vi "Move_Piezo.vi"(5 "Piezo":u16(ring)=1 items=["X (AO0)", "Y (AO1)", "Z (AO2)", "V (AO3)", "V2 (AO4)"], 7 "Movement Speed (µm/s)":dbl=5.0 min=0.0 max=20.0, 11 "Position (µm) (or V)":dbl min=-10.0 max=1000.0) -> ()   [LabVIEW 2023]
uses:
  Sub_Vi/TypeDefs/Settings.ctl
  Sub_Vi/TypeDefs/WayPointCluster.ctl
  Sub_Vi/TypeDefs/ChangeOnFly.ctl
  Settings.vi
panel:
  in  "stop":bool
  in  "WayPointCluster":T1
  in  "SettingsCluster":T2={"Sample Rate (us)"=1, "Samples Per Data Point (int, power of 2)"=1000, "DistanceToBulk (um)"=-1.0, "HoldTimeScaler"=1, "SaveData"=FALSE, "DistanceToBulk (um) 2"=-1.0, "DistanceToBulk (um) 3"=-1.0}
  # "Settings"
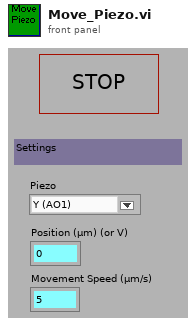
[diagram p1: front panel]
types:
  T1 = typedef "WayPointCluster.ctl" = cluster{"X (um)":dbl[], "Y (um)":dbl[], "Z (um)":dbl[], "V (V)":dbl[], "X Velocity (um s-1)":dbl[], "Y Velocity (um s-1)":dbl[], "Z Velocity (um s-1)":dbl[], "V Velocity (V s-1)":dbl[], "FeedBack Type (enum)":u16[], "Move X (boolean)":bool[], "Move Y (boolean)":bool[], "Move Z (boolean)":bool[], "Move V (boolean)":bool[], "Jump V (boolean)":bool[], "Hold (boolean)":bool[], "Hold Time":u32[], "V2 (V)":dbl[], "Move V2":bool[], "V2 Velocity (V s-1)":dbl[], "Jump V2 (boolean)":bool[], "Update z Position delta (ms)":i16[], "Hold Feedback1":bool[], "Move Z PicoMotor":bool[], " Z PicoMotor Direction":bool[], "DIO0":bool[]}
  T2 = typedef "Settings.ctl" = cluster{"Sample Rate (us)":u32, "Samples Per Data Point (int, power of 2)":i16, "DistanceToBulk (um)":dbl, "HoldTimeScaler":u64, "SaveData":bool, "DistanceToBulk (um) 2":dbl, "DistanceToBulk (um) 3":dbl}
  T3 = typedef "ChangeOnFly.ctl" = cluster{"Stop (boolean)":refnum<vi>, "Pause (boolean)":refnum<vi>, "EndCurrentLine (boolean)":refnum<vi>, "max movement per update step (Interger, nm)":refnum<vi>, "P (float, arb)":refnum<vi>, "Feedback set point (double, Amps)":refnum<vi>, "Voltage (double, V)":refnum<vi>, "Feedback set point 2 (double, Amps)":refnum<vi>, "Stop on Greater Than 2? (boolean)":refnum<vi>, "Stop on Greater Than? (boolean)":refnum<vi>, "Voltage 2 (double, V)":refnum<vi>, "Feedback Type (enum)":refnum<vi>, "Feedback Type 2 (enum)":refnum<vi>}
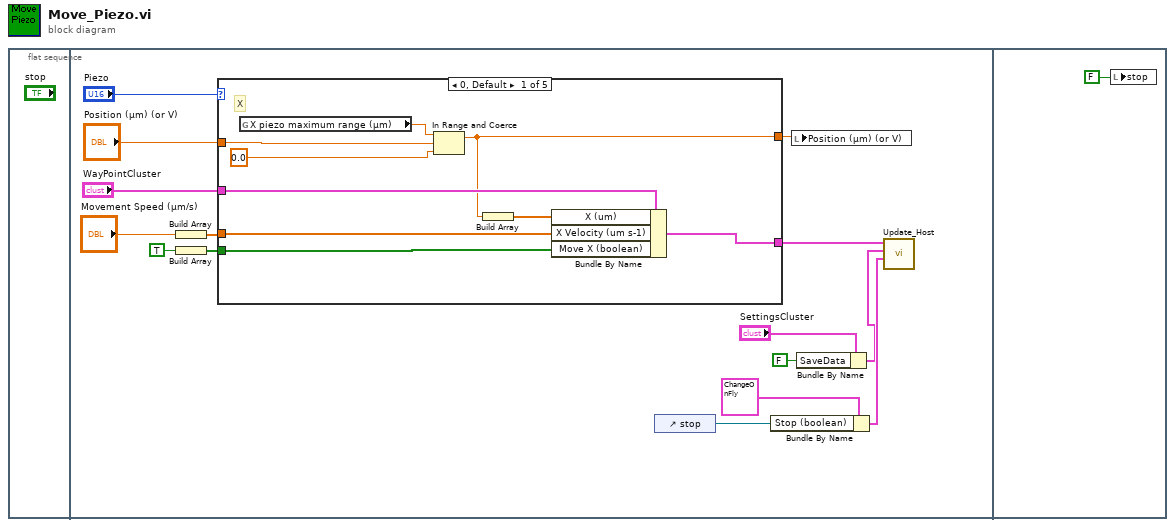
[diagram p0: block diagram]
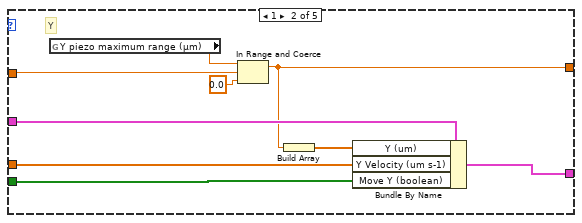
[diagram p2: hidden frame]
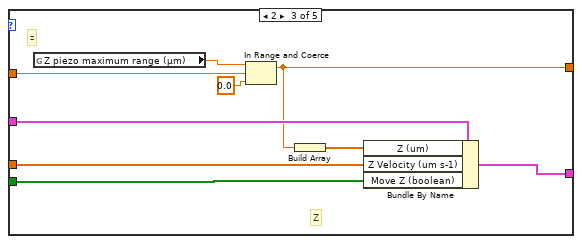
[diagram p3: hidden frame]
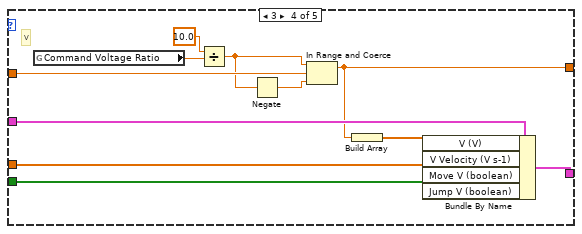
[diagram p4: hidden frame]
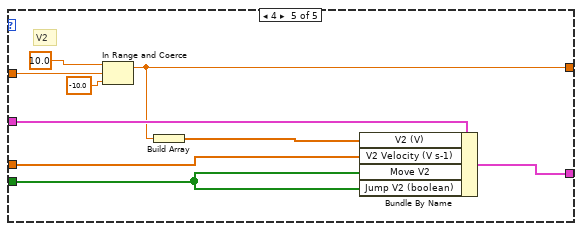
[diagram p5: hidden frame]
diagram:
  n1 = flat-sequence {
    frame #0 {
    }
    frame #1 {
      n2 = Build Array("Movement Speed (µm/s)") -> (w13:dbl[])
      n3 = Build Array(TRUE) -> (w10:bool[])
      n4 = case shown="0, Default" "Piezo" {
        tunnel: "WayPointCluster" -> [w24 w33 w41 w53 w62]
        tunnel: w13 -> [w23 w32 w42 w52 w61]
        tunnel: [w22 w31 w40 w51 w60] -> w7
        tunnel: w10 -> [w21 w30 w39 w47 w59]
        tunnel: "Position (µm) (or V)" -> [w18 w27 w36 w50 w56]
        tunnel: [w17 w26 w35 w49 w55] -> w8
        frame 0, Default {
          # "X"
          n5 = global read "Settings.vi" "X piezo maximum range (µm)"() -> (w19:dbl)
          n6 = In Range and Coerce(upper limit=w19, x=w18, lower limit=0.0) -> (coerced(x)=w17:dbl)  [unwired: 1 out]
          n7 = Build Array(w17) -> (w16:dbl[])
          n8 = Bundle By Name(cluster=w24, "X (um)"=w16, "X Velocity (um s-1)"=w23, "Move X (boolean)"=w21) -> (w22:T1)
        }
        frame 1 {
          # "Y"
          n9 = global read "Settings.vi" "Y piezo maximum range (µm)"() -> (w28:dbl)
          n10 = In Range and Coerce(upper limit=w28, x=w27, lower limit=0.0) -> (coerced(x)=w26:dbl)  [unwired: 1 out]
          n11 = Build Array(w26) -> (w25:dbl[])
          n12 = Bundle By Name(cluster=w33, "Y (um)"=w25, "Y Velocity (um s-1)"=w32, "Move Y (boolean)"=w30) -> (w31:T1)
        }
        frame 2 {
          # "z"
          # "Z"
          n13 = global read "Settings.vi" "Z piezo maximum range (µm)"() -> (w37:dbl)
          n14 = In Range and Coerce(upper limit=w37, x=w36, lower limit=0.0) -> (coerced(x)=w35:dbl)  [unwired: 1 out]
          n15 = Build Array(w35) -> (w34:dbl[])
          n16 = Bundle By Name(cluster=w41, "Z (um)"=w34, "Z Velocity (um s-1)"=w42, "Move Z (boolean)"=w39) -> (w40:T1)
        }
        frame 3 {
          # "V"
          n17 = global read "Settings.vi" "Command Voltage Ratio"() -> (w43:dbl)
          n18 = Divide(x=10.0 ("lower limit"), y=w43) -> (x/y=w44:dbl)
          n19 = Negate(x=w44) -> (-x=w45:dbl)
          n20 = In Range and Coerce(upper limit=w44, x=w50, lower limit=w45) -> (coerced(x)=w49:dbl)  [unwired: 1 out]
          n21 = Build Array(w49) -> (w48:dbl[])
          n22 = Bundle By Name(cluster=w53, "V (V)"=w48, "V Velocity (V s-1)"=w52, "Move V (boolean)"=w47, "Jump V (boolean)"=w47) -> (w51:T1)
        }
        frame 4 {
          # "V2"
          n23 = In Range and Coerce(upper limit=10.0 ("lower limit"), x=w56, lower limit=-10.0) -> (coerced(x)=w55:dbl)  [unwired: 1 out]
          n24 = Build Array(w55) -> (w54:dbl[])
          n25 = Bundle By Name(cluster=w62, "V2 (V)"=w54, "V2 Velocity (V s-1)"=w61, "Move V2"=w59, "Jump V2 (boolean)"=w59) -> (w60:T1)
        }
      }
      n26 = control-ref of="stop"() -> (w6:refnum<vi>)
      n27 = Bundle By Name(cluster=T3 {"Stop (boolean)"=refnum, "Pause (boolean)"=refnum, "EndCurrentLine (boolean)"=refnum, "max movement per update step (Interger, nm)"=refnum, "P (float, arb)"=refnum, "Feedback set point (double, Amps)"=refnum, "Voltage (double, V)"=refnum, "Feedback set point 2 (double, Amps)"=refnum, "Stop on Greater Than 2? (boolean)"=refnum, "Stop on Greater Than? (boolean)"=refnum, "Voltage 2 (double, V)"=refnum, "Feedback Type (enum)"=refnum, "Feedback Type 2 (enum)"=refnum} ("ChangeonFly"), "Stop (boolean)"=w6) -> (w5:T3)
      n28 = local write "Position (µm) (or V)"(w8) -> ()
      n29 = Bundle By Name(cluster="SettingsCluster", "SaveData"=FALSE) -> (w2:T2)
      n30 = call "Update_Host.vi"("ChangeonFly"=w5, "SettingsCluster"=w2, "WayPointCluster"=w7) -> ()  [unwired: 7 in]
    }
    frame #2 {
      n31 = local write "stop"(FALSE) -> ()
    }
  }
